vi "solar_msg Q EnQ.vi"(4 "CMD_DATA Array":variant[](array[variant]), 6 "CMD Array":string[](array[string]), 7 "Priority (Normal)":enum8{"Normal", "Priority", "IgnoreIfExists"}(ring), 8 "error in (no error)":errorcluster, 9 "CMD_DATA (Last)":variant, 10 "CMD (Last)":string, 11 "Queue in":refnum<queue>) -> (0 "error out":errorcluster, 1 "Timed Out?":bool, 3 "Queue out":refnum<queue>)   [LabVIEW 2018]
doc: "This enqueues a message to the queue. The <b>CMD Array</b> is enqueued before the <b>CMD (Last)</b> message. Set the <b>Priority</b> to enqueue to the back (Normal), front (Priority) or filtered (Ignore If Exists)."
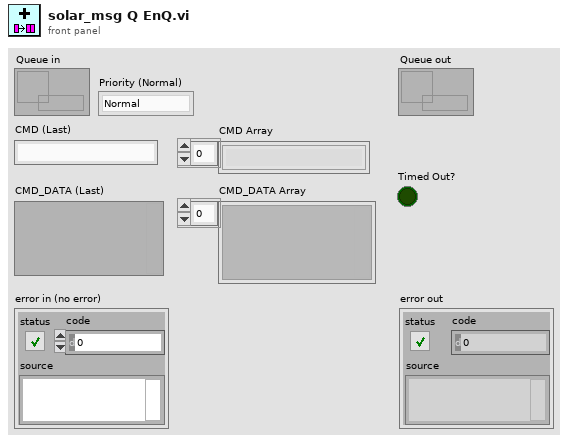
[diagram p1: front panel]
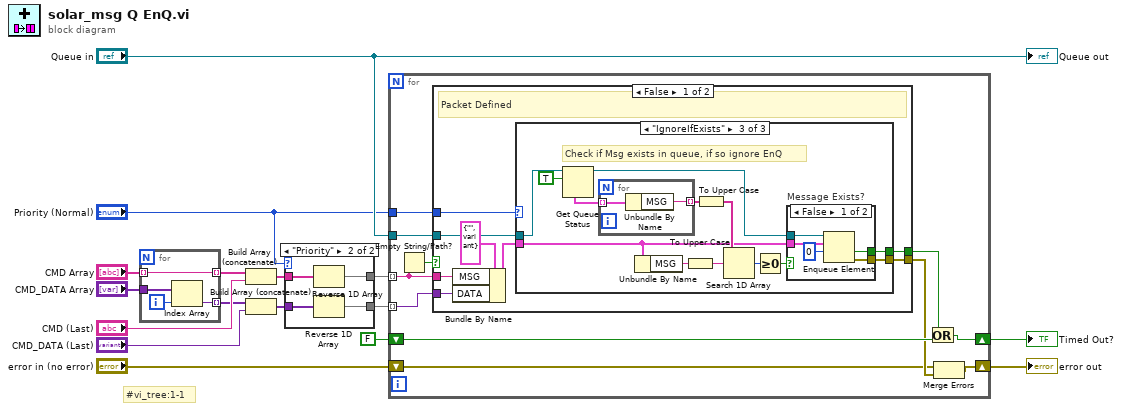
[diagram p0: block diagram]
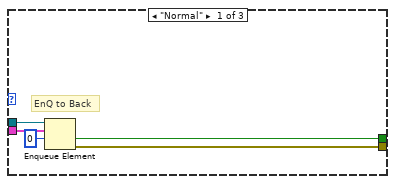
[diagram p3: hidden frame]
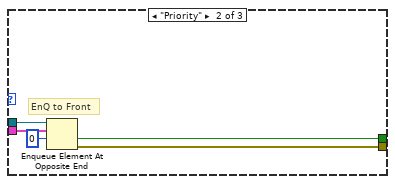
[diagram p4: hidden frame]
diagram:
  # "#vi_tree:1-1"
  n1 = for {
    tunnel: "CMD_DATA Array" -> [w19]
    tunnel: "CMD Array" -> [w18] mode=indexing
    tunnel: [w18] -> w10 mode=indexing
    tunnel: [w17] -> w9 mode=indexing
    i -> [w20]
    n2 = Index Array(array=w19, index=w20) -> (element=w17:variant)
  }
  n3 = Build Array (concatenate)(w10, "CMD (Last)") -> (w14:string[])
  n4 = Build Array (concatenate)(w9, "CMD_DATA (Last)") -> (w13:variant[])
  n5 = case shown="\"Priority\"" "Priority (Normal)" {
    tunnel: w14 -> [w22 w26]
    tunnel: w13 -> [w21 w25]
    tunnel: [w22 w24] -> w7
    tunnel: [w21 w23] -> w6
    frame Default {
    }
    frame "Priority" {
      n6 = Reverse 1D Array(array=w26) -> (reversed array=w24:string[])
      n7 = Reverse 1D Array(array=w25) -> (reversed array=w23:variant[])
    }
  }
  n8 = for {
    tunnel: "Priority (Normal)" -> [w29]
    tunnel: w7 -> [w28] mode=indexing
    tunnel: w6 -> [w27] mode=indexing
    shift-right: [w32] -> w3
    shift-left: "error in (no error)" -> [w33]
    shift-right: [w37] -> w2
    shift-left: FALSE -> [w36]
    tunnel: "Queue in" -> [w30]
    n9 = Empty String/Path?(string/path=w28) -> (empty?=w35:bool)
    n10 = case shown="False" w35 {
      tunnel: [w45 _] -> w34
      tunnel: w30 -> [w44 _]
      tunnel: w29 -> [w43 _]
      tunnel: w28 -> [w39 _]
      tunnel: [w42 _] -> w31
      tunnel: w27 -> [w38 _]
      frame False {
        # "Packet Defined"
        n11 = Bundle By Name(cluster=cluster{"MSG":string, "DATA":variant} {"MSG"="", "DATA"=variant} ("PACKET"), "MSG"=w39, "DATA"=w38) -> (w40:cluster{"MSG":string, "DATA":variant})
        n12 = case shown="\"IgnoreIfExists\"" w43 {
          tunnel: w44 -> [w50 w55 w68]
          tunnel: [w48 w51 w66] -> w42
          tunnel: w40 -> [w47 w53 w57]
          tunnel: [w49 w54 w67] -> w45
          frame "Normal" {
            # "EnQ to Back"
            n13 = Enqueue Element(queue=w50, element=w47, timeout in ms (-1)=0) -> (timed out?=w48:bool, error out=w49:errorcluster)  [unwired: 1 in, 1 out]
          }
          frame "Priority" {
            # "EnQ to Front"
            n14 = Enqueue Element At Opposite End(queue=w55, element=w53, timeout in ms (-1)=0) -> (timed out?=w51:bool, error out=w54:errorcluster)  [unwired: 1 in, 1 out]
          }
          frame "IgnoreIfExists" {
            # "Check if Msg exists in queue, if so ignore EnQ"
            n15 = Get Queue Status(queue=w68, return elements? (F)=TRUE) -> (queue out=w64:refnum<queue>, elements=w61:cluster{"MSG":string, "DATA":variant}[])  [unwired: 1 in, 6 out]
            n16 = for {
              tunnel: w61 -> [w70] mode=indexing
              tunnel: [w69] -> w60 mode=indexing
              n17 = Unbundle By Name(w70) -> ("MSG"=w69:string)
            }
            n18 = Unbundle By Name(w57) -> ("MSG"=w56:string)
            n19 = To Upper Case(1:w56) -> (0:w58:string)
            n20 = To Upper Case(1:w60) -> (0:w59:string[])
            n21 = Search 1D Array(1D array=w59, element=w58) -> (index of element=w63:i32)  [unwired: 1 in]
            n22 = Greater Or Equal To 0?(x=w63) -> (x >= 0?=w62:bool)
            n23 = case "Message Exists?" shown="False" w62 {
              tunnel: [w75 _] -> w67
              tunnel: [w71 _] -> w66
              tunnel: w64 -> [w73 _]
              tunnel: w57 -> [w72 _]
              frame False {
                n24 = Enqueue Element(queue=w73, element=w72, timeout in ms (-1)=0) -> (timed out?=w71:bool, error out=w75:errorcluster)  [unwired: 1 in, 1 out]
              }
              frame True {
              }
            }
          }
        }
      }
      frame True {
        # "Empty Packet"
      }
    }
    n25 = Or(x=w31, y=w36) -> (x .or. y?=w37:bool)
    n26 = Merge Errors(w33, w34) -> (w32:errorcluster)
  }
  "error out" <- w3
  "Timed Out?" <- w2
  "Queue out" <- "Queue in"
